vi "SubVI_SendTime.vi"(11 "mqtt prefix":string="test/example") -> ()   [LabVIEW 2017]
uses:
  Global mqttExample.vi
  mqtt-LabVIEW/src/class/mqtt/mqtt.lvclass
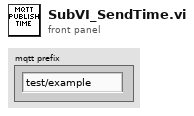
[diagram p1: front panel]
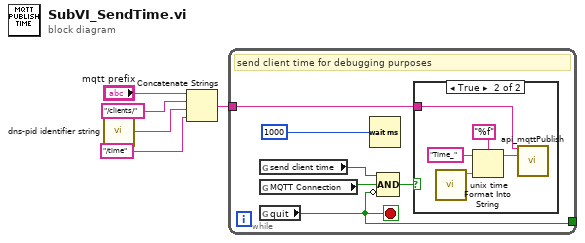
[diagram p0: block diagram]
diagram:
  n1 = call "dns-pid identifier string.vi"() -> ("DNS_PID Identifier string"=w4:string)  [unwired: 1 in]
  n2 = Concatenate Strings("mqtt prefix", "/clients/" ("string"), w4, "/time" ("string")) -> (w2:string)
  n3 = while {
    tunnel: w2 -> [w9]
    tunnel: [w8] -> _
    stop <- w8 stop-if-true
    # "send client time for debugging purposes"
    n4 = global read "Global mqttExample.vi" "send client time"() -> (w6:bool)
    n5 = global read "Global mqttExample.vi" "MQTT Connection"() -> (w7:bool)
    n6 = global read "Global mqttExample.vi" "quit"() -> (w8:bool)
    n7 = Wait (ms)(milliseconds to wait=u32 1000) -> ()  [unwired: 1 out]
    n8 = Compound Arithmetic op=AND(w6, w7, invert w8) -> (w10:bool)
    n9 = case shown="True" w10 {
      tunnel: w9 -> [_ w13]
      frame False {
      }
      frame True {
        n10 = call "unix time.vi"() -> ("Unix time"=w15:dbl)  [unwired: 10 in, 1 out]
        n11 = Format Into String(format string="%f", initial string="Time_", w15) -> (resulting string=w14:string)  [unwired: 1 in, 1 out]
        n12 = call "api_mqttPublish.vi"("topic"=w13, "value"=w14) -> ()  [unwired: 12 in, 2 out]
      }
    }
  }
